vi "veclen.vi"(5 "Overwrite Lib Path":path, 8 "error in (no error)":errorcluster, 11 "index_ptr":u64) -> (0 "error out":errorcluster, 2 "Vector Length":u32, 3 "index_ptr out":u64)   [LabVIEW 2020, in "KD Tree.lvlib"]
doc: "FLANN_EXPORT unsigned int flann_veclen(flann_index_t index_ptr);"
uses:
  KD Tree.lvlib
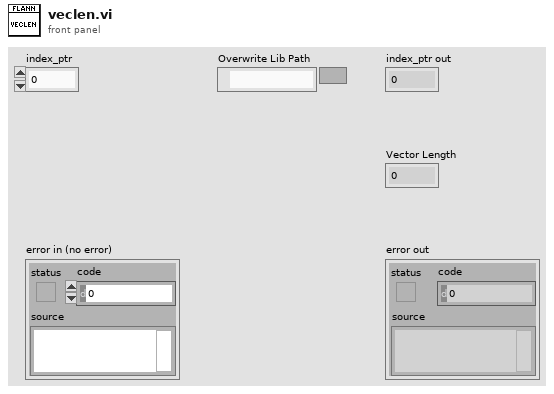
[diagram p1: front panel]
types:
  T1 = typedef "Semaphore RefNum" = refnum<k1>
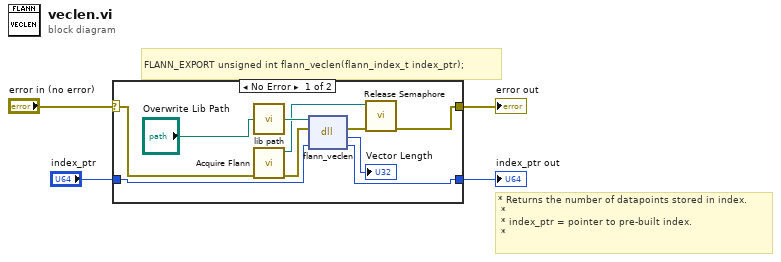
[diagram p0: block diagram]
diagram:
  # "* Returns the number of datapoints stored in index.\n *\n * index_ptr = pointer to pre-built index.\n *"
  # "FLANN_EXPORT unsigned int flann_veclen(flann_index_t index_ptr);"
  n1 = case shown="No Error" "error in (no error)" {
    selector: "error in (no error)" -> [w12 w16]
    tunnel: "index_ptr" -> [w14 w15]
    tunnel: [w13 w15] -> w3
    tunnel: [w6 w16] -> w1
    frame No Error {
      n2 = call "lib path.vi"("Overwrite Lib Path"="Overwrite Lib Path") -> ("lib path"=w10:path)
      n3 = call "Acquire Flann.vi"("error in (no error)"=w12) -> ("error out"=w7:errorcluster, "semaphore"=w5:T1)  [unwired: 9 in]
      n4 = dll-call lib="E:/Labview/LV 2020/Libs/flann/flann.*" fn="flann_veclen"(path in=w10, error in=w7, "index_ptr"=w14) -> (error out=w11:errorcluster, "return type"=→"Vector Length":u32, "index_ptr"=w13:u64)  [unwired: 1 in, 1 out]
      n5 = call <vilib>:"Release Semaphore.vi"("error in (no error)"=w11, "semaphore"=w5) -> ("error out"=w6:errorcluster)  [unwired: 4 in, 1 out]
    }
    frame Error {
    }
  }
  "index_ptr out" <- w3
  "error out" <- w1
